vi "GetPositionData.vi"(0 "object in":refnum<class "Battleship.lvclass">, 5 "error in (no error)":errorcluster) -> (14 "object out":refnum<class "Battleship.lvclass">, 15 "Footprint":bool[][](array[boolean]), 16 "MapPositions":T1[](array[typedef]), 17 "HitPositions":T1[](array[typedef]), 19 "error out":errorcluster)   [LabVIEW 2015, in "Battleship.lvclass"]
uses:
  Battleship.lvclass
  TypDefs/Coordinates.ctl
  Battleship.lvclass/Battleship.ctl
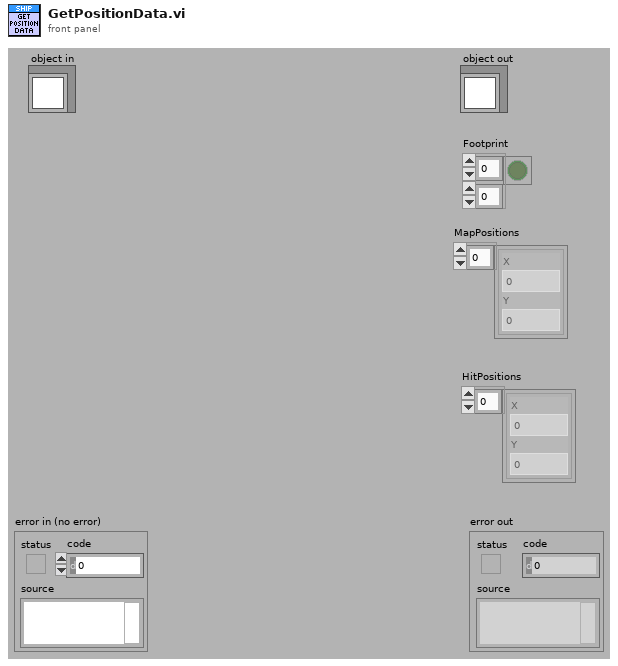
[diagram p1: front panel]
types:
  T1 = typedef "Coordinates.ctl" = cluster{"X":i32, "Y":i32}
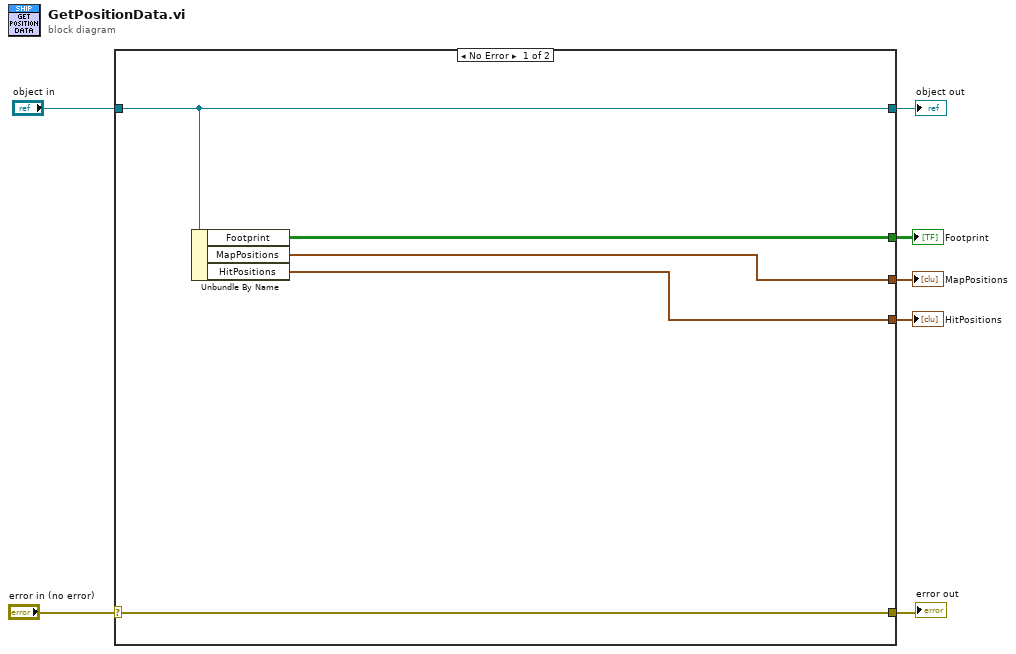
[diagram p0: block diagram]
diagram:
  n1 = case shown="No Error" "error in (no error)" {
    selector: "error in (no error)" -> [w12 w14]
    tunnel: [w12 w14] -> w6
    tunnel: [w11 w13] -> w4
    tunnel: "object in" -> [w11 w13]
    tunnel: [w10 _] -> w3
    tunnel: [w9 _] -> w2
    tunnel: [w8 _] -> w1
    frame No Error {
      n2 = Unbundle By Name(w11) -> ("Footprint"=w10:bool[][], "MapPositions"=w9:T1[], "HitPositions"=w8:T1[])
    }
    frame Error {
    }
  }
  "error out" <- w6
  "object out" <- w4
  "Footprint" <- w3
  "MapPositions" <- w2
  "HitPositions" <- w1
